vi "Netburner_RD_Loop2.vi"(0 "VISA resource name (COM Port #)":refnum<visa-resource-name>="COM3", 2 "Mode (0)":i32, 3 "Error In (no error)":errorcluster, 4 "Wait (sec)":dbl=5.0) -> (1 "#  Bytes Read":u32=207, 5 "Return String from Device":string="Waiting 2sec to start 'A' to abort\r\nConfigured IP = 0.0.0.0\r\nConfigured Mask = 0.0.0.0\r\nMAC Address= 00:03:f4:07:76:b7\r\n\r\n AD5754 SPI DAC Test Routine \r\nEnter the DAC number (0-3) and value (-10. to 10.): \r\n", 6 "Error Out":errorcluster={"status"=FALSE, "code"=1073676294, "source"="VISA Read in Galvant_GPIB_RD_Loop.vi"})   [LabVIEW 2013]
uses:
  <vilib>/Instr/_visa.llb/VISA Configure Serial Port (Instr).vi
  Instance           3 34Saved   Prologix LabVIEW 7 Example .vi
panel:
  out "Examples":string="Useful strings:\n+test\n+a:10\nID?"
  # "Netburner Read Loop VI"
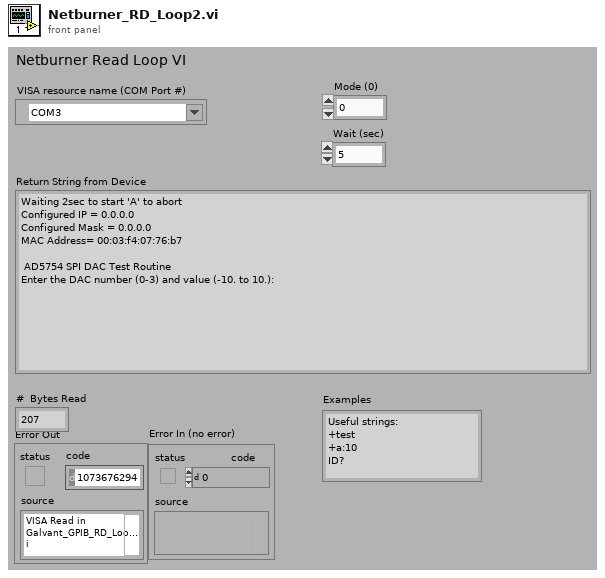
[diagram p1: front panel]
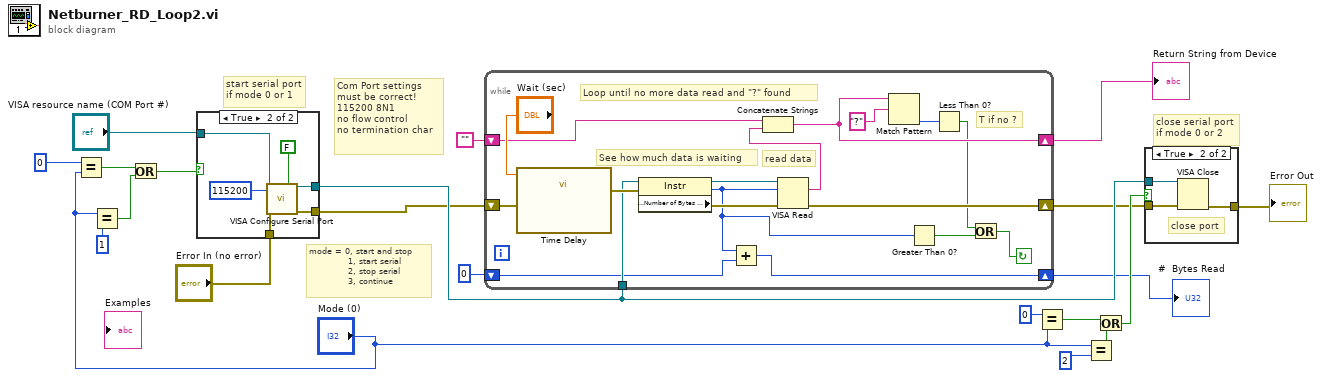
[diagram p0: block diagram]
diagram:
  # "mode = 0, start and stop\n             1, start serial\n             2, stop serial\n             3, continue"
  # "Com Port settings\nmust be correct!\n115200 8N1\nno flow control\nno termination char"
  # "close serial port\nif mode 0 or 2"
  # "start serial port\nif mode 0 or 1"
  n1 = Equal?(x=0, y="Mode (0)") -> (x = y?=w12:bool)
  n2 = Equal?(x="Mode (0)", y=1) -> (x = y?=w10:bool)
  n3 = Or(x=w12, y=w10) -> (x .or. y?=w11:bool)
  n4 = case shown="True" w11 {
    tunnel: "VISA resource name (COM Port #)" -> [w23 w29]
    tunnel: [w23 w28] -> w7
    tunnel: [w22 w27] -> w4
    tunnel: "Error In (no error)" -> [w22 w24]
    frame False {
    }
    frame True {
      n5 = call-poly "VISA Configure Serial Port"("VISA resource name"=w29, "Enable Termination\nChar (T)"=FALSE, "baud rate (9600)"=115200, "error in (no error)"=w24) -> ("VISA resource name out"=w28:refnum<visa-resource-name>, "error out"=w27:errorcluster)  [unwired: 10 in]
    }
  }
  n6 = while {
    tunnel: w7 -> [w44]
    shift-right: [w35] -> w5
    shift-left: "" -> [w42]
    shift-right: [w39] -> w3
    shift-left: w4 -> [w41]
    shift-right: [w36] -> w1
    shift-left: 0 -> [w37]
    stop <- w30 continue-if-true
    # "T if no ?"
    # "Loop until no more data read and \"?\" found"
    # "read data"
    # "See how much data is waiting"
    n7 = call "Time Delay"("error in (no error)"=w41, "Delay Time (s)"="Wait (sec)") -> ("error out"=w46:errorcluster)  [unwired: 9 in]
    n8 = property class="Instr"(reference=w44, error in=w46) -> (reference out=w45:refnum<visa-resource-name>, error out=w40:errorcluster, "Serial Settings:Number of Bytes at Serial Port"=w38:u32)
    n9 = Add(x=w38, y=w37) -> (x+y=w36:u32)
    n10 = VISA Read(VISA resource name=w45, byte count=w38, error in (no error)=w40) -> (read buffer=w43:string, error out=w39:errorcluster)  [unwired: 2 out]
    n11 = Concatenate Strings "Concatenate Strings"(w42, w43) -> (w35:string)
    n12 = Match Pattern(string=w35, regular expression="?") -> (offset past match=w33:i32)  [unwired: 1 in, 3 out]
    n13 = Greater Than 0?(x=w38) -> (x > 0?=w32:bool)
    n14 = Less Than 0?(x=w33) -> (x < 0?=w31:bool)
    n15 = Or(x=w31, y=w32) -> (x .or. y?=w30:bool)
  }
  "Return String from Device" <- w5
  "#  Bytes Read" <- w1
  n16 = Equal?(x=0, y="Mode (0)") -> (x = y?=w16:bool)
  n17 = Equal?(x="Mode (0)", y=2) -> (x = y?=w14:bool)
  n18 = Or(x=w16, y=w14) -> (x .or. y?=w13:bool)
  n19 = case shown="True" w13 {
    tunnel: w7 -> [_ w51]
    tunnel: w3 -> [w48 w50]
    tunnel: [w48 w49] -> w20
    frame False {
    }
    frame True {
      # "close port"
      n20 = VISA Close(VISA resource name=w51, error in (no error)=w50) -> (error out=w49:errorcluster)
    }
  }
  "Error Out" <- w20
